vi "PWM_Motor_Folgen.vi"(0 "Geschw_IR_vorne":dbl, 1 "Geschwindigkeit\nmultiplikator":dbl) -> (7 "PWM Lenkung":dbl)   [LabVIEW 2016]
uses:
  <vilib>/addons/control/pid/pid.llb/PID (DBL).vi
  <vilib>/addons/control/pid/NI_PID_pid.lvlib
panel:
  in  "PID gains":T1={"proportional gain (Kc)"=1.0, "integral time (Ti, min)"=0.01, "derivative time (Td, min)"=0.0} {"derivative time (Td, min)" format="%.3f"; "integral time (Ti, min)" format="%.3f"; "proportional gain (Kc)" format="%.3f"}
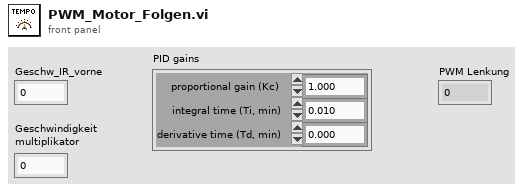
[diagram p1: front panel]
types:
  T1 = cluster{"proportional gain (Kc)":dbl, "integral time (Ti, min)":dbl, "derivative time (Td, min)":dbl}
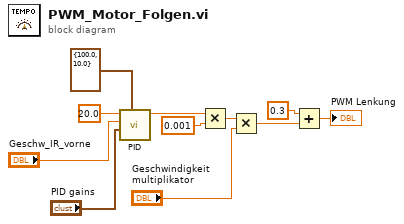
[diagram p0: block diagram]
diagram:
  n1 = call-poly <vilib>:"PID.vi"("output range"=cluster{"output high":dbl, "output low":dbl} {"output high"=100.0, "output low"=10.0}, "PID gains"="PID gains", "process variable"="Geschw_IR_vorne", "setpoint"=20.0) -> ("output"=w7:dbl)  [unwired: 6 in, 1 out]
  n2 = Multiply(x=w7, y=0.001) -> (x*y=w3:dbl)
  n3 = Multiply(x=w3, y="Geschwindigkeit\nmultiplikator") -> (x*y=w2:dbl)
  n4 = Add(x=0.3, y=w2) -> (x+y=→"PWM Lenkung":dbl)
